vi "writeToXML.vi"(8 "error in (no error)":errorcluster, 10 "ClassLabel":string, 11 "AbsorbOffset in":refnum<class "AbsorbOffset.lvclass">) -> (0 "error out":errorcluster, 2 "XML out":string, 3 "AbsorbOffset out":refnum<class "AbsorbOffset.lvclass">)   [LabVIEW 2014, in "TCSDataDefinitions.lvlib" / "TCSCommand.lvlib" / "OffsetCommands.lvlib" / "AbsorbOffset.lvclass"]
uses:
  AbsorbOffset.lvclass
  AbsorbOffset.lvclass/AbsorbOffset.ctl
  TargetOffsetCommands/TargetOffsetCommands.lvclass
  <userlib>/Common/XML/XMLGenerator/XMLGenerator.lvclass
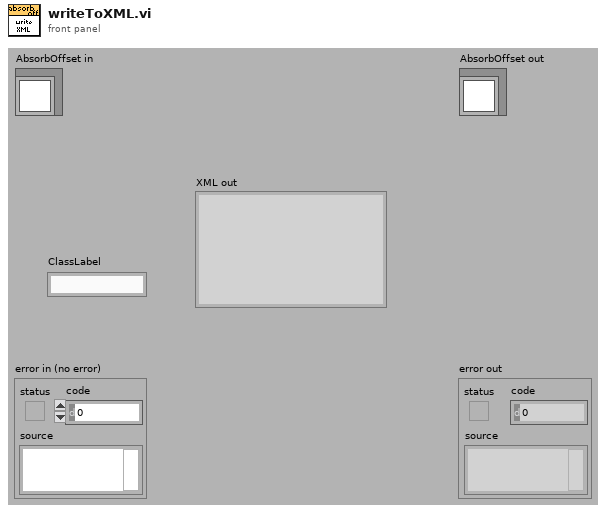
[diagram p1: front panel]
types:
  T1 = typedef "TCSDataDefinitions.lvlib/TCSCommand.lvlib/OffsetCommands.lvlib/Num2Types.ctl" = enum16{"User", "Handset", "Both"}
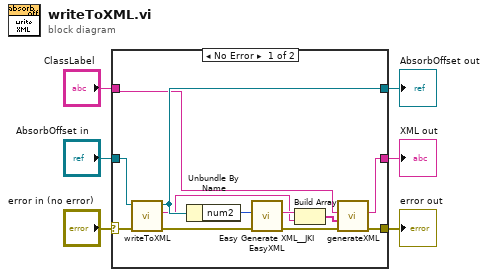
[diagram p0: block diagram]
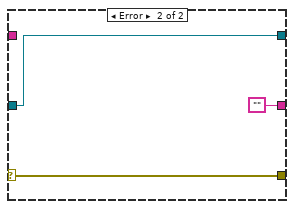
[diagram p2: hidden frame]
diagram:
  n1 = case shown="No Error" "error in (no error)" {
    selector: "error in (no error)" -> [w10 w21]
    tunnel: [w14 w21] -> w5
    tunnel: [w11 w20] -> w3
    tunnel: "AbsorbOffset in" -> [w12 w20]
    tunnel: [w13 ""] -> w2
    tunnel: "ClassLabel" -> [w8 _]
    frame No Error {
      n2 = call-parent "writeToXML.vi"("error in (no error)"=w10, "TargetOffsetCommands in"=w12) -> ("error out"=w9:errorcluster, "XML out"=w7:string, "TargetOffsetCommands out"=w11:refnum<class "AbsorbOffset.lvclass">)  [unwired: 7 in]
      n3 = Unbundle By Name(w11) -> ("num2"=w18:T1)
      n4 = call <vilib>:"Easy Generate XML__JKI EasyXML.vi"("error in (no error)"=w9, "LabVIEW Data"=w18) -> ("error out"=w15:errorcluster, "XML String"=w16:string)  [unwired: 8 in]
      n5 = Build Array(w16, w7) -> (w17:string[])
      n6 = call <userlib>:"generateXML.vi"("error in"=w15, "childrenXML"=w17, "elementName"=w8) -> ("error out"=w14:errorcluster, "XML out"=w13:string)  [unwired: 6 in, 1 out]
    }
    frame Error {
    }
  }
  "error out" <- w5
  "AbsorbOffset out" <- w3
  "XML out" <- w2
